vi "Configuration.Free.Writer.Test.vi"() -> ()   [LabVIEW 2017, in "Measurement.Free.lvclass"]
uses:
  Measurement.Free.lvclass
  Typedefs/Configuration--Cluster.ctl
  Typedefs/Configuration.Hardware--Cluster.ctl
  Measurement/Typedefs/Configuration.SMU--Cluster.ctl
  SMU/Typedefs/Configuration--Cluster.ctl
  Measurement/Typedefs/Configuration.LIA--Cluster.ctl
  LIA/Typedefs/Configuration--Cluster.ctl
  Measurement/Typedefs/Configuration.OPM--Cluster.ctl
  OPM/Typedefs/Configuration--Cluster.ctl
  Measurement/Typedefs/Configuration.OPA--Cluster.ctl
  OPA/Typedefs/Configuration--Cluster.ctl
  <vilib>/Utility/config.llb/NI_LVConfig.lvlib
  SMU/SMU.lvclass
  Measurement/Measurement.lvclass
  LIA/LIA.lvclass
  OPM/OPM.lvclass
  OPA/OPA.lvclass
panel:
  in  "Configuration.Free":T1={"Measurement.Type"=enum."Free", "Hardware"={"SMU"={"Enable"=TRUE, "SMU Model"="Keithley2600", "Configuration"={"VISA Resource"="GPIB0::26::INSTR", "Channel"="A"}}, "LIA"={"Enable"=TRUE, "LIA Model"="SR810", "Configuration"={"VISA Resource"="GPIB0::8::INSTR"}}, "OPM"={"Enable"=TRUE, "OPM Model"="ThorlabsPM400", "Configuration"={"VISA Resource"="USB0::0x1313::0x8075::P5001221::INSTR"}}, "OPA"={"Enable"=TRUE, "OPA Model"="OrpheusHP", "Configuration"={"Serial Number"="Orpheus-HP-Demo-8047"}}}}
  out "error out":errorcluster
  # "e"
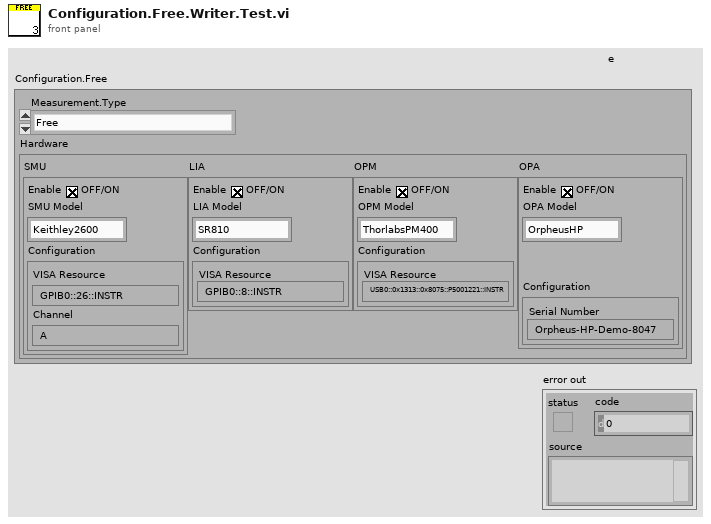
[diagram p1: front panel]
types:
  T1 = typedef "Measurement.Free.lvclass/Configuration--Cluster.ctl" = cluster{"Measurement.Type":enum16{"Free", "I/V Curve", "Wavelength sweeping", "Photocurrent mapping"}, "Hardware":T2}
  T2 = typedef "Measurement.Free.lvclass/Configuration.Hardware--Cluster.ctl" = cluster{"SMU":T3, "LIA":T5, "OPM":T7, "OPA":T9}
  T3 = typedef "Measurement.lvclass/Configuration.SMU--Cluster.ctl" = cluster{"Enable":bool, "SMU Model":string, "Configuration":T4}
  T4 = typedef "SMU.lvclass/Configuration--Cluster.ctl" = cluster{"VISA Resource":string, "Channel":string}
  T5 = typedef "Measurement.lvclass/Configuration.LIA--Cluster.ctl" = cluster{"Enable":bool, "LIA Model":string, "Configuration":T6}
  T6 = typedef "LIA.lvclass/Configuration--Cluster.ctl" = cluster{"VISA Resource":string}
  T7 = typedef "Measurement.lvclass/Configuration.OPM--Cluster.ctl" = cluster{"Enable":bool, "OPM Model":string, "Configuration":T8}
  T8 = typedef "OPM.lvclass/Configuration--Cluster.ctl" = cluster{"VISA Resource":string}
  T9 = typedef "Measurement.lvclass/Configuration.OPA--Cluster.ctl" = cluster{"Enable":bool, "OPA Model":string, "Configuration":T10}
  T10 = typedef "OPA.lvclass/Configuration--Cluster.ctl" = cluster{"Serial Number":string}
  T11 = typedef "NI_LVConfig.lvlib/Config Data RefNum.ctl" = refnum<k1>
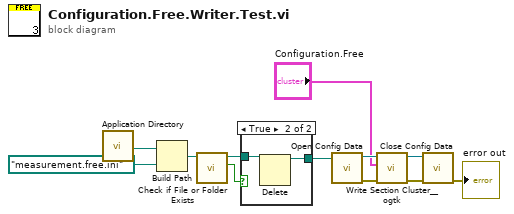
[diagram p0: block diagram]
diagram:
  n1 = call <vilib>:"Application Directory.vi"() -> ("Application Directory"=w12:path)
  n2 = Build Path(base path=w12, name or relative path=path "measurement.free.ini") -> (appended path=w1:path)
  n3 = call <vilib>:"Check if File or Folder Exists.vi"("path"=w1) -> ("file or folder exists?"=w3:bool, "dup path"=w4:path)  [unwired: 8 in, 1 out]
  n4 = case shown="True" w3 {
    tunnel: [w13 w15] -> w2
    tunnel: w4 -> [w13 w14]
    frame False {
    }
    frame True {
      n5 = Delete(path (use dialog)=w14) -> (deleted path=w15:path)  [unwired: 4 in, 2 out]
    }
  }
  n6 = call <vilib>:"Open Config Data.vi"("configuration file path"=w2) -> ("error out"=w10:errorcluster, "refnum"=w7:T11)  [unwired: 8 in, 1 out]
  n7 = call <userlib>:"Write Section Cluster__ogtk.vi"("error in (no error)"=w10, "Section Formatted Cluster"="Configuration.Free", "refnum"=w7) -> ("error out"=w9:errorcluster, "dup refnum"=w8:T11)  [unwired: 7 in]
  n8 = call <vilib>:"Close Config Data.vi"("error in (no error)"=w9, "refnum"=w8) -> ("error out"=→"error out":errorcluster)  [unwired: 8 in, 1 out]
